vi "Create SV.vi"(4 "custom control":variant, 6 "data type":T1(ring)=enum."double", 7 "Mode (commit)":u16(ring) items=["commit", "buffer"], 8 "Error In":errorcluster, 9 "shared variable name":string, 10 "process name":string, 11 "CS++DSCManager in":refnum<class "CS++DSCManager.lvclass">) -> (0 "Error Out":errorcluster, 1 "Shared Variable":refnum<k21>, 3 "CS++DSCManager out":refnum<class "CS++DSCManager.lvclass">)   [LabVIEW 2016, in "CS++DSCManager.lvlib" / "CS++DSCManager.lvclass"]
doc: "Creates a shared variable of the given name and type in the specified process. The shared variable that you want to create replaces an existing shared variable if the two shared variables have the same name."
uses:
  CS++DSCManager.lvclass
  <vilib>/lvdsc/NI_DSC.lvlib
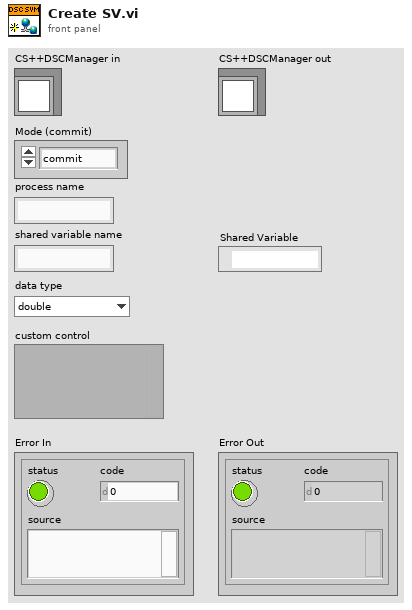
[diagram p1: front panel]
types:
  T1 = enum32{"u32BitField", "bool", "double", "string", "int8", "uint8", "int16", "uint16", "int32", "uint32", "int64", "uint64", "single", "double waveform", "int16 waveform", "array of boolean", "array of int8", "array of uint8", "array of int16", "array of uint16", "array of int32", "array of uint32", "array of int64", "array of uint64", "array of single", "array of double", "array of double waveform", "array of int16 waveform", "array of string", "variant", "timestamp", "fixed point", "custom"}
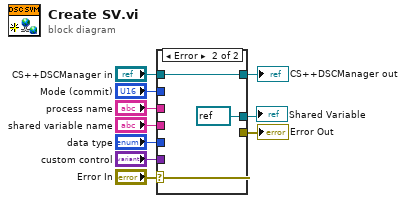
[diagram p0: block diagram]
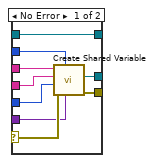
[diagram p2: hidden frame]
diagram:
  n1 = case shown="Error" "Error In" {
    selector: "Error In" -> [w18 w22]
    tunnel: [w17 w22] -> w9
    tunnel: [w19 w21] -> w7
    tunnel: "CS++DSCManager in" -> [w19 w21]
    tunnel: "process name" -> [w16 _]
    tunnel: "Mode (commit)" -> [w15 _]
    tunnel: "shared variable name" -> [w14 _]
    tunnel: "data type" -> [w13 _]
    tunnel: "custom control" -> [w12 _]
    tunnel: [w11 refnum<k21> refnum ("shared variable")] -> w1
    frame No Error {
      n2 = call <vilib>:"Create Shared Variable.vi"("custom control"=w12, "set mode"=w15, "error in (no error)"=w18, "data type"=w13, "shared variable name"=w14, "process name"=w16) -> ("error out"=w17:errorcluster, "shared variable"=w11:refnum<k21>)  [unwired: 3 in, 1 out]
    }
    frame Error {
    }
  }
  "Error Out" <- w9
  "CS++DSCManager out" <- w7
  "Shared Variable" <- w1
